vi "多参数数据插入.vi"(8 "error in (no error)":errorcluster caption="错误输入（无错误）", 9 "编号":string, 10 "columns enable":T1, 11 "data in":T2) -> (0 "error out":errorcluster)   [LabVIEW 2016, in "斯坦道多参数.lvlib"]
uses:
  <vilib>/Utility/sysdir.llb/System Directory Type.ctl
  <vilib>/addons/database/Auxilliary.llb/DB Tools Parameter Info.ctl
  <vilib>/addons/database/Auxilliary.llb/DB Tools DataTypes.ctl
  <vilib>/addons/database/Auxilliary.llb/DB Tools Parameter Dir.ctl
  <vilib>/addons/database/Auxilliary.llb/DB Tools Column Info.ctl
  <vilib>/addons/database/Auxilliary.llb/DB Tools Format Datetime String (Time Stamp).vi
  <vilib>/addons/database/Connection.llb/DB Tools Open Connec (String).vi
  <vilib>/addons/database/Connection.llb/Conn Execute.vi
  <vilib>/addons/database/Recordset.llb/Rec Destroy - Connection.vi
  <vilib>/addons/database/Command.llb/Cmd Set Parameter Value (C).vi
  <vilib>/addons/database/Command.llb/Cmd Execute.vi
  <vilib>/addons/database/Recordset.llb/Rec Destroy - Command.vi
  <vilib>/addons/database/Command.llb/Cmd Delete.vi
  <vilib>/addons/database/NI_Database_API.lvlib
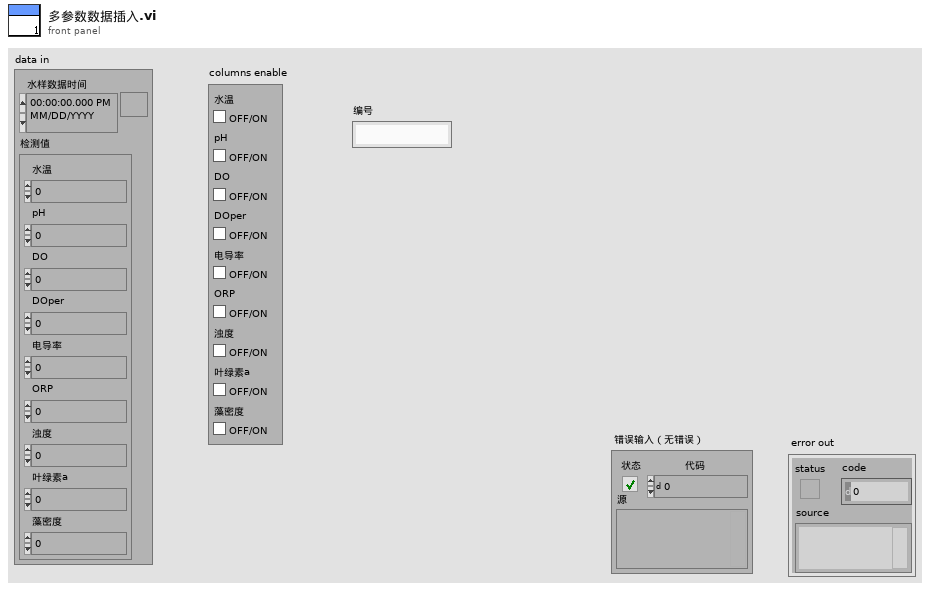
[diagram p1: front panel]
types:
  T1 = cluster{"水温":bool, "pH":bool, "DO":bool, "DOper":bool, "电导率":bool, "ORP":bool, "浊度":bool, "叶绿素a":bool, "藻密度":bool}
  T2 = cluster{"水样数据时间":timestamp, "检测值":cluster{"水温":dbl, "pH":dbl, "DO":dbl, "DOper":dbl, "电导率":dbl, "ORP":dbl, "浊度":dbl, "叶绿素a":dbl, "藻密度":dbl}}
  T3 = typedef "System Directory Type.ctl" = i32
  T4 = cluster{"水温":dbl, "pH":dbl, "DO":dbl, "DOper":dbl, "电导率":dbl, "ORP":dbl, "浊度":dbl, "叶绿素a":dbl, "藻密度":dbl}
  T5 = typedef "NI_Database_API.lvlib/DB Tools Column Info.ctl" = cluster{"column name":string, "data type":T6, "size":i32, "allow null?":bool}
  T6 = typedef "NI_Database_API.lvlib/DB Tools DataTypes.ctl" = enum16{"String", "Long (I32)", "Single (SGL)", "Double (DBL)", "Date/Time", "Binary"}
  T7 = typedef "NI_Database_API.lvlib/DB Tools Parameter Info.ctl" = cluster{"parameter name":string, "type":T6, "direction":T8, "value":variant}
  T8 = typedef "NI_Database_API.lvlib/DB Tools Parameter Dir.ctl" = enum32{"Input", "Output", "Input/Output", "Return Value"}
  T9 = typedef "NI_Database_API.lvlib/Conn ObjectReference.ctl" = refnum<k1>
  T10 = typedef "NI_Database_API.lvlib/Rec ObjectReference.ctl" = refnum<k1>
  T11 = typedef "NI_Database_API.lvlib/Cmd ObjectReference.ctl" = refnum<k1>
  T12 = typedef "NI_Database_API.lvlib/Cmd-Rec Object Reference.ctl" = refnum<k1>
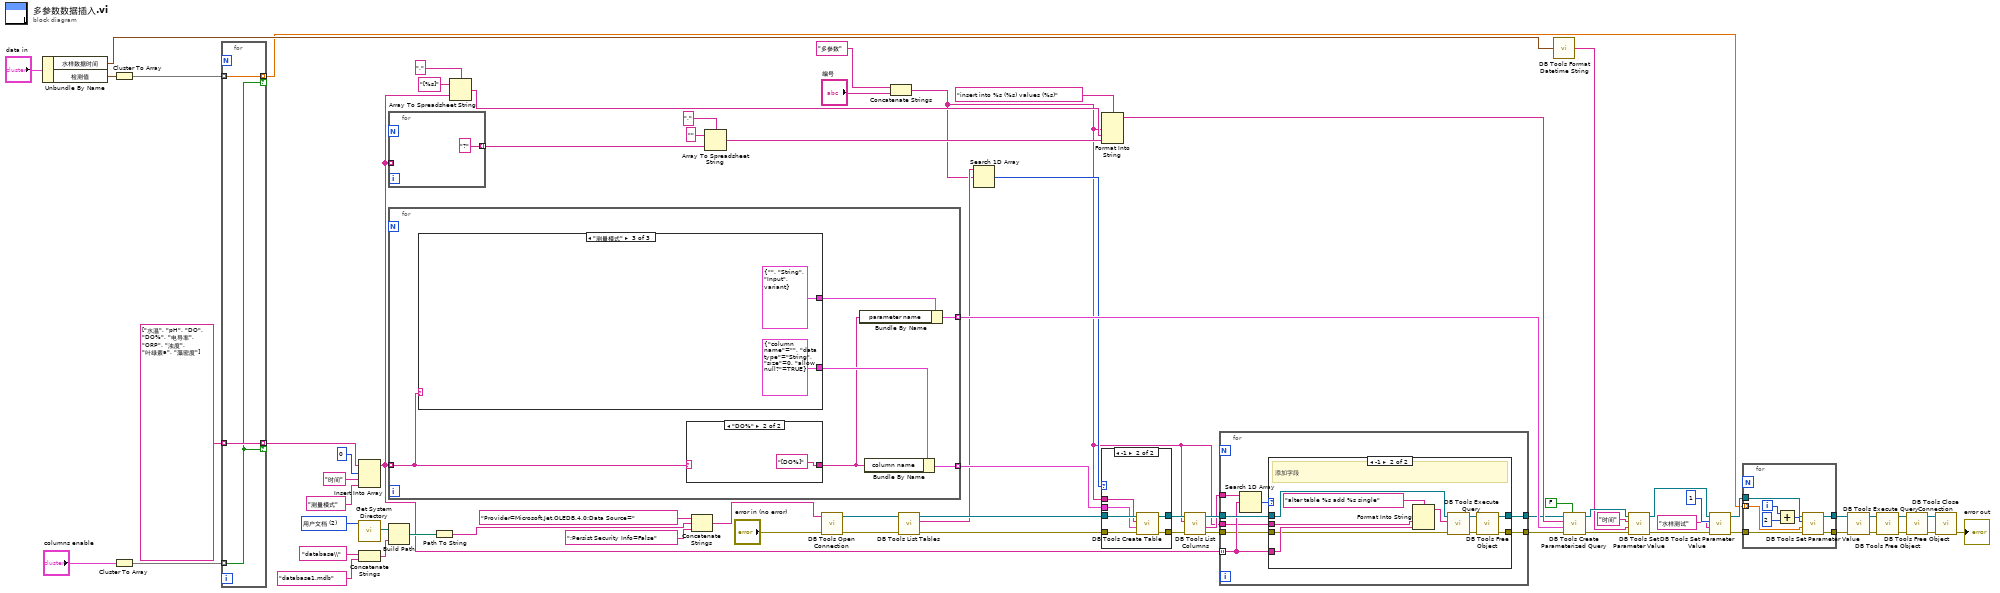
[diagram p0: block diagram]
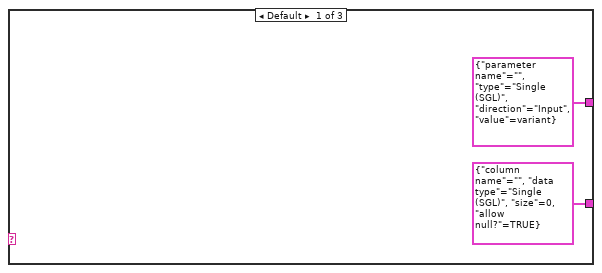
[diagram p5: hidden frame]
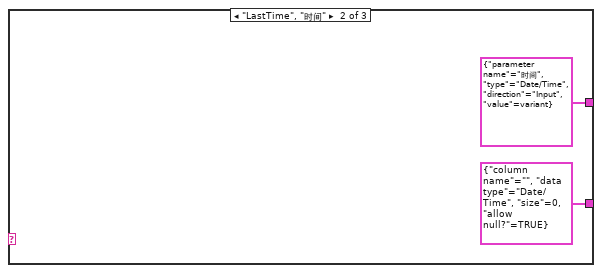
[diagram p6: hidden frame]
diagram:
  w71 = T3 2 items=["用户目录"=0, "用户桌面"=1, "用户文档"=2, "用户应用程序数据"=3, "用户设置"=4, "用户临时目录"=5, "公共文档"=6, "公共应用程序数据"=7, "公共设置"=8, "公共缓存"=13, "系统核心库"=9, "系统安装库"=10, "应用程序文件"=11, "启动盘根目录"=12] ("system directory type")
  n1 = Unbundle By Name("data in") -> ("水样数据时间"=w27:timestamp, "检测值"=w17:T4)
  n2 = Cluster To Array(cluster=w17) -> (array=w16:dbl[])
  n3 = Cluster To Array(cluster="columns enable") -> (array=w55:bool[])
  n4 = for {
    tunnel: string[] ["水温", "pH", "DO", "DO%", "电导率", "ORP", "浊度", "叶绿素a", "藻密度"] ("columns name") -> [w74] mode=indexing
    tunnel: w55 -> [w72] mode=indexing
    tunnel: [w74] -> w4 mode=indexing if=w72
    tunnel: w16 -> [w73] mode=indexing
    tunnel: [w73] -> w15 mode=indexing if=w72
  }
  n5 = Insert Into Array(array=w4, index=0 ("索引"), new element #1="时间" ("新元素/子数组"), new element #2="测量模式" ("新元素/子数组")) -> (w12:string[])
  n6 = call <vilib>:"Get System Directory.vi"("system directory type"=w71) -> ("system directory"=w69:path)  [unwired: 10 in]
  n7 = Concatenate Strings("database\\" ("condition"), "database1.mdb" ("字符串")) -> (w63:string)
  n8 = for {
    tunnel: w12 -> [_] mode=indexing
    tunnel: ["?"] -> w42 mode=indexing
  }
  n9 = for {
    tunnel: w12 -> [w77] mode=indexing
    tunnel: [w78] -> w40 mode=indexing
    tunnel: [w80] -> w39 mode=indexing
    n10 = case shown="\"测量模式\"" w77 {
      tunnel: [T7 {"parameter name"="", "type"=enum."Single (SGL)", "direction"=enum."Input", "value"=variant} ("parameter information") T7 {"parameter name"="时间", "type"=enum."Date/Time", "direction"=enum."Input", "value"=variant} ("parameter information") T7 {"parameter name"="", "type"=enum."String", "direction"=enum."Input", "value"=variant} ("parameter information")] -> w79
      tunnel: [T5 {"column name"="", "data type"=enum."Single (SGL)", "size"=0, "allow null?"=TRUE} ("column information") T5 {"column name"="", "data type"=enum."Date/Time", "size"=0, "allow null?"=TRUE} ("column information") T5 {"column name"="", "data type"=enum."String", "size"=0, "allow null?"=TRUE} ("column information")] -> w81
      frame Default {
      }
      frame "LastTime", "时间" {
      }
      frame "测量模式" {
      }
    }
    n11 = case shown="\"DO%\"" w77 {
      selector: w77 -> [w82 _]
      tunnel: [w82 "[DO%]"] -> w76
      frame "假", Default {
      }
      frame "DO%" {
      }
    }
    n12 = Bundle By Name(cluster=w79, "parameter name"=w76) -> (w78:T7)
    n13 = Bundle By Name(cluster=w81, "column name"=w76) -> (w80:T5)
  }
  n14 = Build Path(base path=w69, name or relative path=w63) -> (appended path=w68:path)
  n15 = Path To String(path=w68) -> (string=w67:string)
  n16 = Array To Spreadsheet String(delimiter (Tab)="," ("分隔符(Tab)"), array=w12, 3:"[%s]" ("格式字符串")) -> (spreadsheet string=w51:string)
  n17 = Concatenate Strings("Provider=Microsoft.Jet.OLEDB.4.0;Data Source=" ("condition"), w67, ";Persist Security Info=False" ("condition")) -> (w65:string)
  n18 = Array To Spreadsheet String(delimiter (Tab)="," ("分隔符(Tab)"), array=w42, 3:"" ("格式字符串")) -> (spreadsheet string=w46:string)
  n19 = call-poly <vilib>:"DB Tools Open Connection.vi"("error in (no error)"="error in (no error)", "connection information"=w65) -> ("error out"=w59:errorcluster, "connection reference"=w61:T9)  [unwired: 6 in]
  n20 = Concatenate Strings("多参数" ("字符串"), "编号") -> (w1:string)
  n21 = call <vilib>:"DB Tools List Tables.vi"("error in (no error)"=w59, "connection reference"=w61) -> ("error out"=w38:errorcluster, "tables"=w36:string[], "connection reference out"=w41:T9)  [unwired: 3 in]
  n22 = Search 1D Array(1D array=w36, element=w1) -> (index of element=w35:i32)  [unwired: 1 in]
  n23 = Format Into String(format string="insert into %s (%s) values (%s)" ("格式字符串"), w1, w51, w46) -> (resulting string=w45:string)  [unwired: 2 in, 1 out]
  n24 = case shown="-1" w35 {
    tunnel: w41 -> [w91 w97]
    tunnel: [w91 w96] -> w11
    tunnel: [w90 w95] -> w9
    tunnel: w39 -> [_ w93]
    tunnel: w38 -> [w90 w94]
    tunnel: w1 -> [_ w92]
    frame 0, Default {
    }
    frame -1 {
      n25 = call <vilib>:"DB Tools Create Table.vi"("error in (no error)"=w94, "column information"=w93, "table"=w92, "connection reference"=w97) -> ("error out"=w95:errorcluster, "connection reference out"=w96:T9)  [unwired: 4 in]
    }
  }
  n26 = call <vilib>:"DB Tools List Columns.vi"("error in (no error)"=w9, "table"=w1, "connection reference"=w11) -> ("error out"=w7:errorcluster, "columns"=w8:string[], "connection reference out"=w10:T9)  [unwired: 1 in, 1 out]
  n27 = for {
    tunnel: w12 -> [w102] mode=indexing
    tunnel: w10 -> [w103]
    tunnel: w8 -> [w105]
    tunnel: w7 -> [w101]
    tunnel: [w100] -> w5
    tunnel: [w99] -> w6
    tunnel: w1 -> [w98]
    n28 = Search 1D Array(1D array=w105, element=w102) -> (index of element=w104:i32)  [unwired: 1 in]
    n29 = case shown="-1" w104 {
      tunnel: [w107 w113] -> w99
      tunnel: [w106 w112] -> w100
      tunnel: w103 -> [w107 w111]
      tunnel: w102 -> [_ w110]
      tunnel: w101 -> [w106 w109]
      tunnel: w98 -> [_ w108]
      frame 0, Default {
      }
      frame -1 {
        # "添加字段"
        n30 = Format Into String(format string="alter table %s add %s single", w108, w110) -> (resulting string=w114:string)  [unwired: 2 in, 1 out]
        n31 = call-poly <vilib>:"DB Tools Execute Query.vi"("error in (no error)"=w109, "SQL query"=w114, "connection reference"=w111) -> ("error out"=w116:errorcluster, "recordset reference"=w117:T10)  [unwired: 5 in]
        n32 = call-poly <vilib>:"DB Tools Free Object.vi"("error in (no error)"=w116, "recordset reference"=w117) -> ("error out"=w112:errorcluster, "connection reference"=w113:T9)  [unwired: 8 in]
      }
    }
  }
  n33 = call-poly <vilib>:"DB Tools Format Datetime String.vi"("time stamp"=w27) -> ("date/time string"=w26:string)
  n34 = call <vilib>:"DB Tools Create Parameterized Query.vi"("auto-detect parameters? (F)"=FALSE, "error in (no error)"=w5, "parameters"=w40, "SQL query"=w45, "connection reference"=w6) -> ("error out"=w44:errorcluster, "command reference"=w43:T11)  [unwired: 2 in, 1 out]
  n35 = call-poly <vilib>:"DB Tools Set Parameter Value.vi"("error in (no error)"=w44, "value"=w26, "parameter index"="时间", "command reference"=w43) -> ("error out"=w23:errorcluster, "command reference out"=w24:T11)  [unwired: 4 in]
  n36 = call-poly <vilib>:"DB Tools Set Parameter Value.vi"("error in (no error)"=w23, "value"="水样测试", "parameter index"=1, "command reference"=w24) -> ("error out"=w18:errorcluster, "command reference out"=w19:T11)  [unwired: 4 in]
  n37 = for {
    tunnel: w19 -> [w121]
    tunnel: w18 -> [w122]
    tunnel: w15 -> [w120] mode=indexing
    tunnel: [w119] -> w14
    tunnel: [w118] -> w13
    i -> [w125]
    n38 = Add(x=w125, y=2) -> (x+y=w123:i32)
    n39 = call-poly <vilib>:"DB Tools Set Parameter Value.vi"("error in (no error)"=w122, "value"=w120, "parameter index"=w123, "command reference"=w121) -> ("error out"=w118:errorcluster, "command reference out"=w119:T11)  [unwired: 4 in]
  }
  n40 = call-poly <vilib>:"DB Tools Execute Query.vi"("error in (no error)"=w13, "command reference"=w14) -> ("error out"=w32:errorcluster, "command-recordset reference"=w33:T12)  [unwired: 6 in]
  n41 = call-poly <vilib>:"DB Tools Free Object.vi"("error in (no error)"=w32, "command-recordset reference"=w33) -> ("error out"=w31:errorcluster, "command reference"=w30:T11)  [unwired: 8 in]
  n42 = call-poly <vilib>:"DB Tools Free Object.vi"("error in (no error)"=w31, "command reference"=w30) -> ("error out"=w28:errorcluster, "connection reference"=w29:T9)  [unwired: 8 in]
  n43 = call <vilib>:"DB Tools Close Connection.vi"("error in (no error)"=w28, "connection reference"=w29) -> ("error out"=→"error out":errorcluster)  [unwired: 5 in]
